vi "MotionProfileGeneratorZeroVelocityPoint.vi"(1 "Filter2Sum":dbl, 2 "Filter1Sum":dbl) -> (0 "Zero Velocity":bool)   [LabVIEW 2018, in "ArgosLib.lvlib"]
uses:
  ArgosLib.lvlib
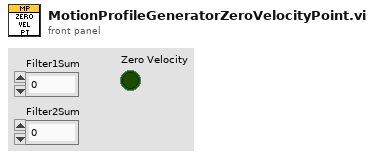
[diagram p1: front panel]
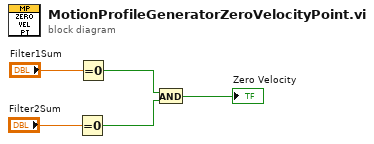
[diagram p0: block diagram]
diagram:
  n1 = Equal To 0?(x="Filter2Sum") -> (x = 0?=w2:bool)
  n2 = Equal To 0?(x="Filter1Sum") -> (x = 0?=w3:bool)
  n3 = And(x=w3, y=w2) -> (x .and. y?=→"Zero Velocity":bool)
